vi "Rig - Editor.vi"(8 "Error IN":errorcluster) -> (0 "error out":errorcluster)   [LabVIEW 2018]
doc: "This VI allows the user to reprocess and reprint data sheets from previously run ESS test. User can search for vibe or thermal test for both actuators and controllers through this portal. Double click serial number from 'Available Data Files' listbox and press 'Print' to initiate report regeneration."
uses:
  controls/Rig Config Settings.ctl
  controls/Command IN_Recipe.ctl
  Globals/Global - Configuration Options.vi
panel:
  in  "Rename":bool
  in  "Exit":bool
  out "Rig Config File Name":string
  in  "Rig Settings":T1={"Rig Name"="", "Rig Room"="1.4", "Base Directory"="", "Computer IP Address"="", "Globals Name"="", "Treatmill Str"="", "cRIO Test Data Dir"=path "", "ai"="", "ao"="", "dio"="", "A_calib_str_row1"="", "A_calib_str_row2"="0", "A_calib_str_row3"="1.4", "Zero_V_str"="", "step_V"="", "Sample Freq"="", "ai_threshold"="", "run_speed_thresh"="", "speed_time_length"="", "wall ball gain"="", "max wall pos"="", "max cor width"="", "Trial Config Directory"=path "C:/Whisker Tester/Trials", "Randomize Trials?"=FALSE}
  in  "Save":bool
  in  "New":bool
  in  "Delete":bool
  in  "Rig File List":i32(listbox)
  in  "Refresh":bool
  out "Rig File Path":path
  in  "Functions":enum16{"Initialize", "Exit"}(ring)
  out "Rig Config Directory":path=path "C:/Data"
  # "Rig Configuration Screen"
  # "*click on rig file to view"
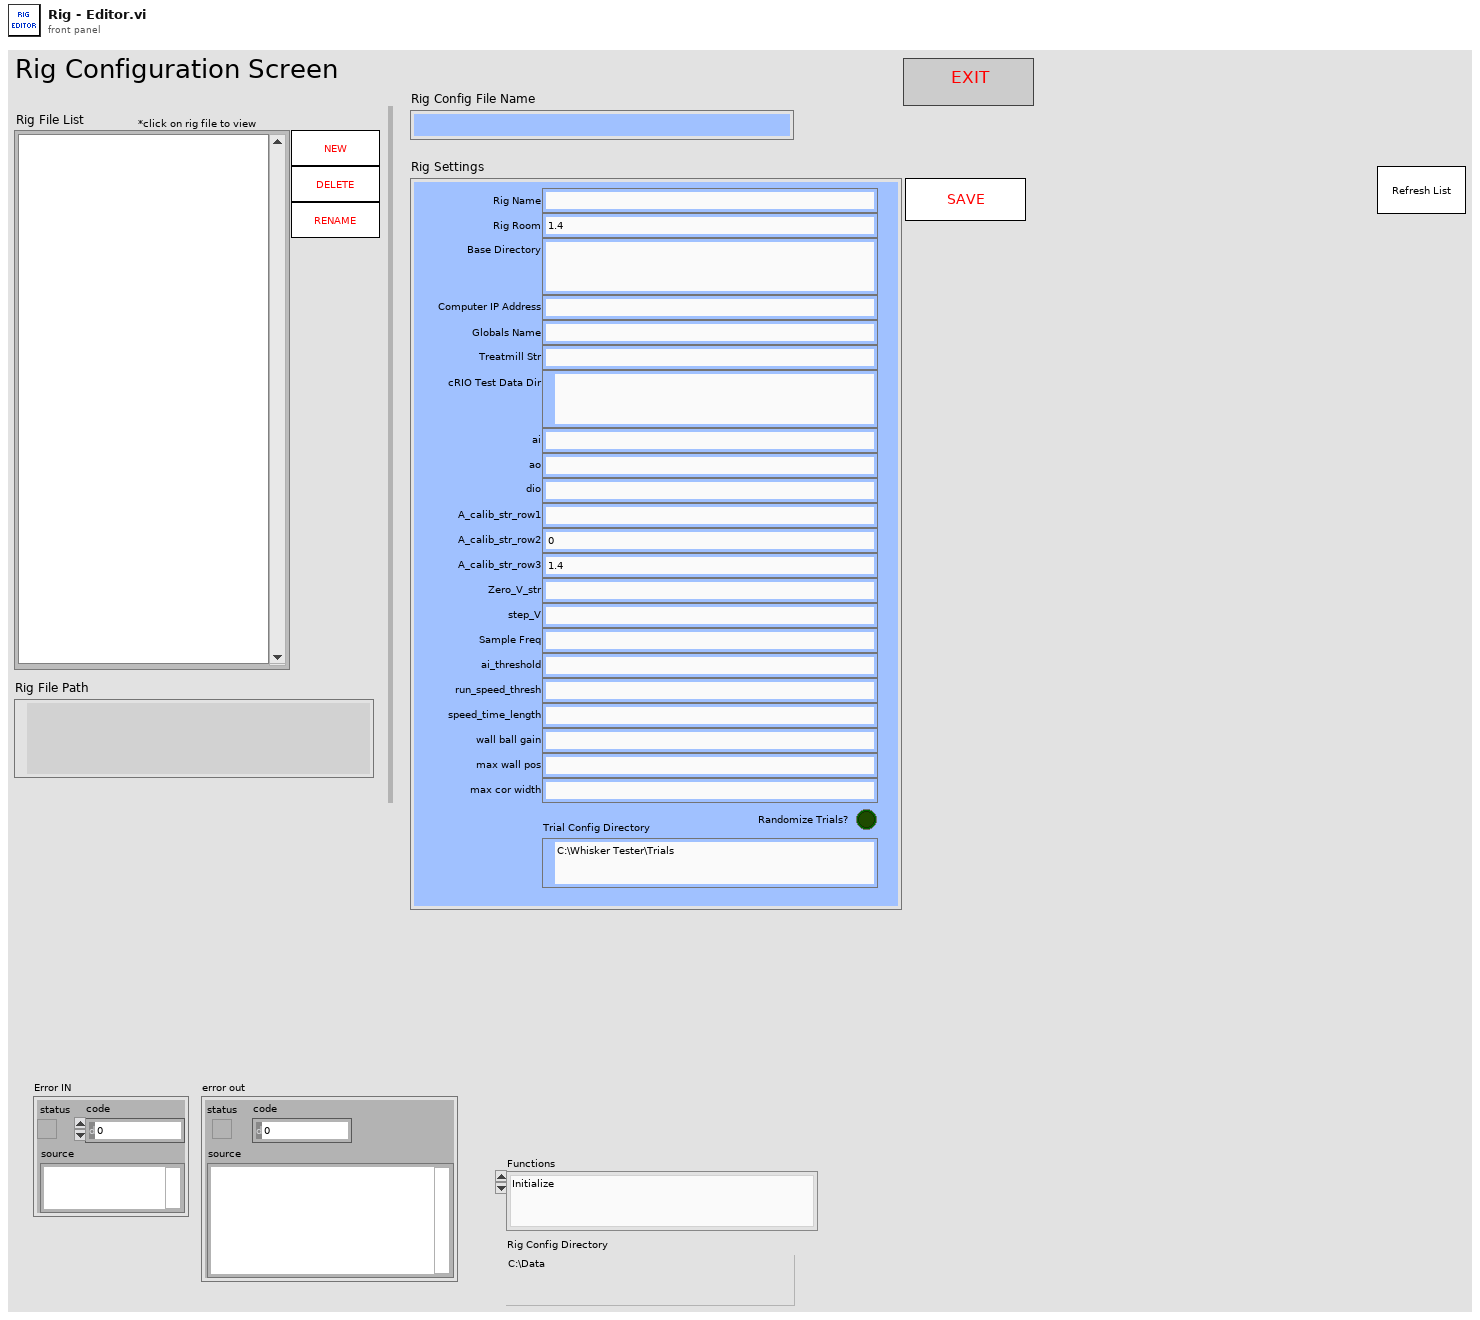
[diagram p1: front panel]
types:
  T1 = typedef "Rig Config Settings.ctl" = cluster{"Rig Name":string, "Rig Room":string, "Base Directory":string, "Computer IP Address":string, "Globals Name":string, "Treatmill Str":string, "cRIO Test Data Dir":path, "ai":string, "ao":string, "dio":string, "A_calib_str_row1":string, "A_calib_str_row2":string, "A_calib_str_row3":string, "Zero_V_str":string, "step_V":string, "Sample Freq":string, "ai_threshold":string, "run_speed_thresh":string, "speed_time_length":string, "wall ball gain":string, "max wall pos":string, "max cor width":string, "Trial Config Directory":path, "Randomize Trials?":bool}
  T2 = typedef "Command IN_Recipe.ctl" = enum16{"Save", "Load"}
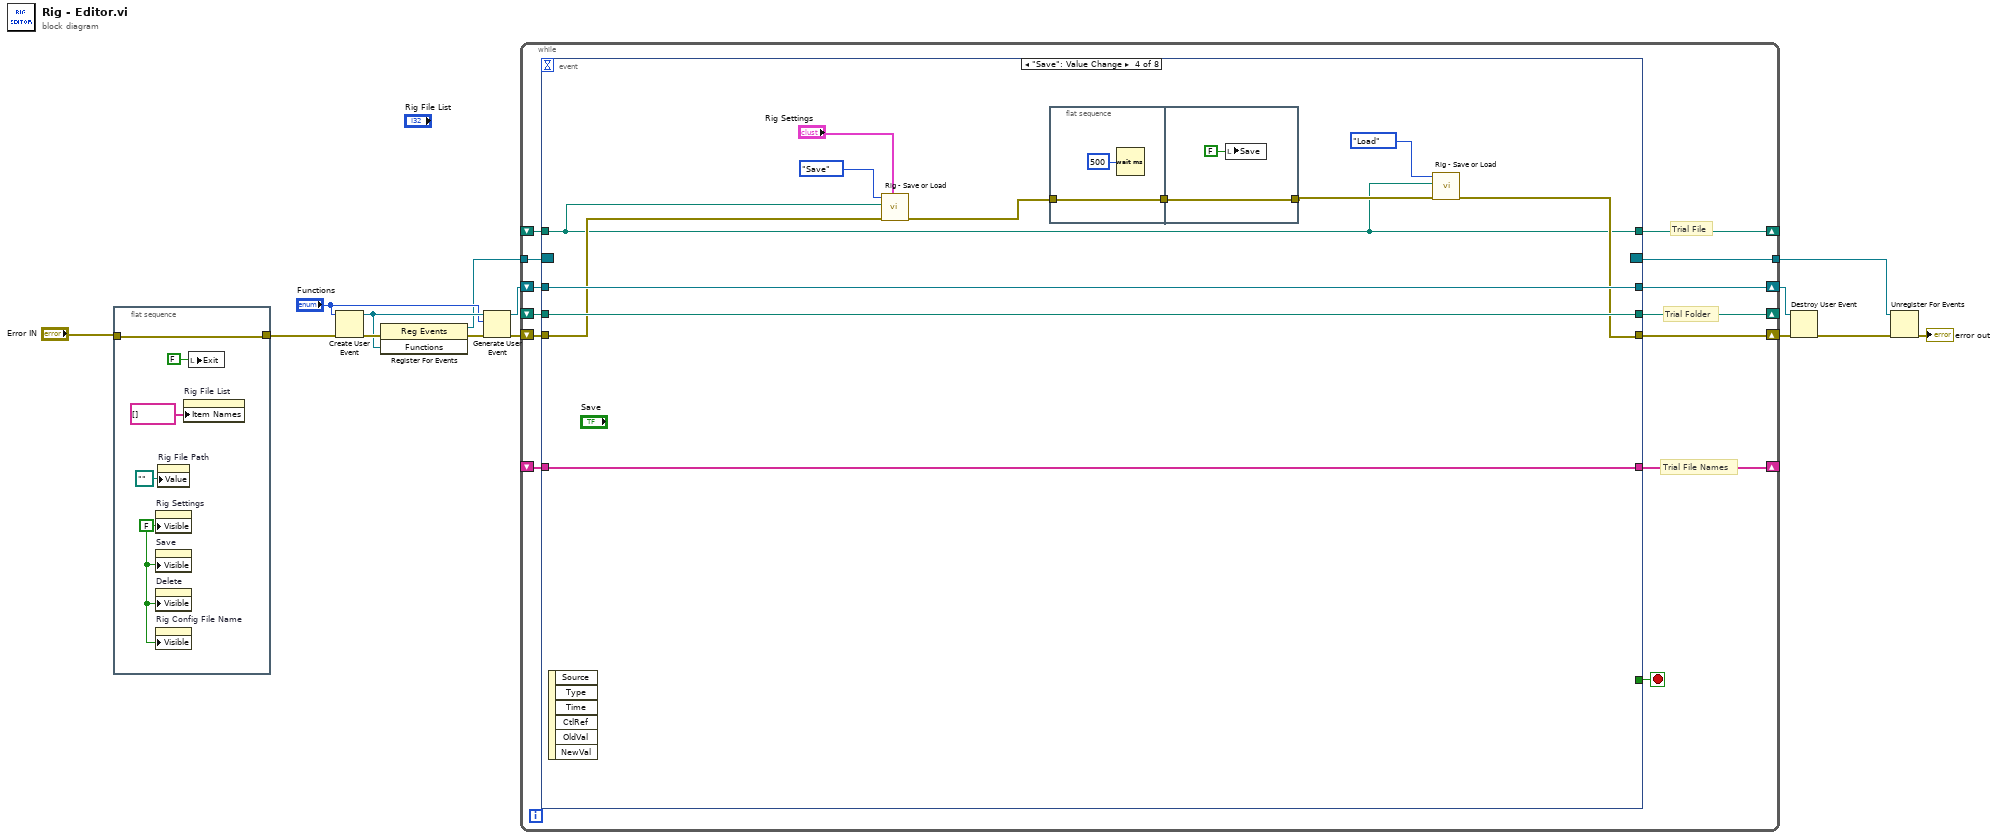
[diagram p0: block diagram]
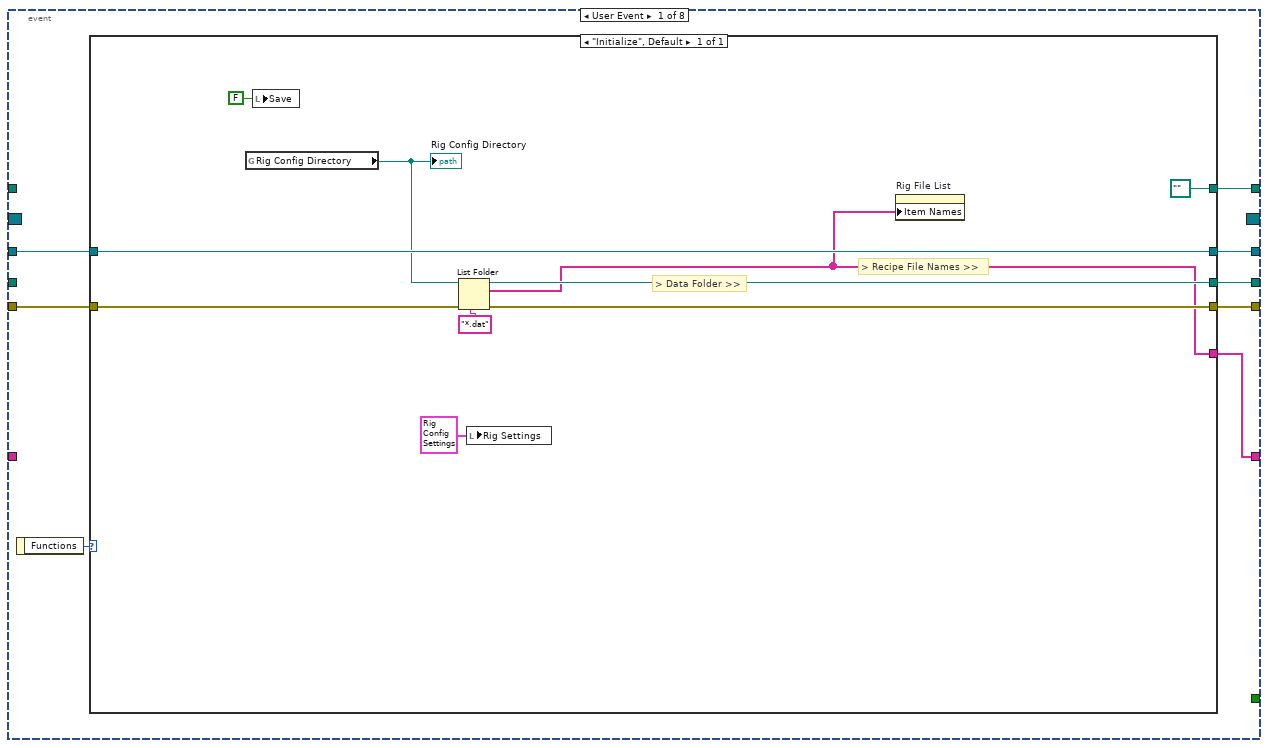
[diagram p2: hidden frame]
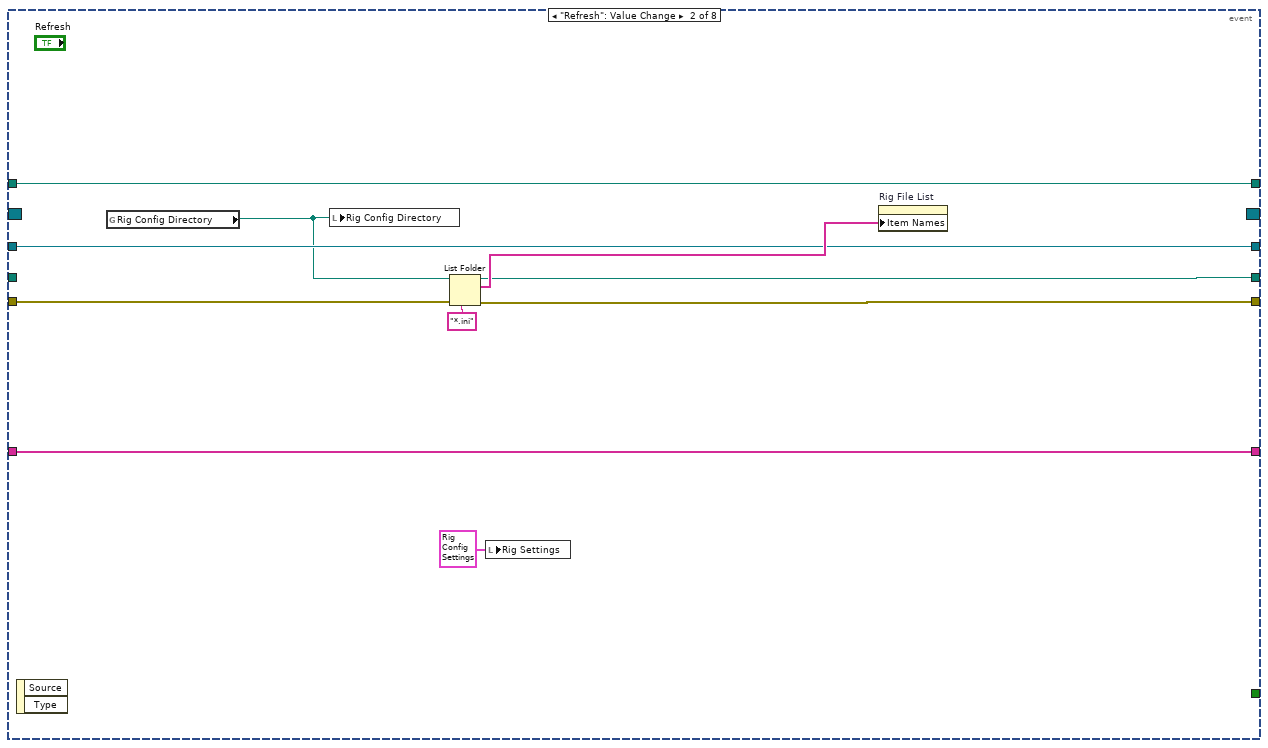
[diagram p3: hidden frame]
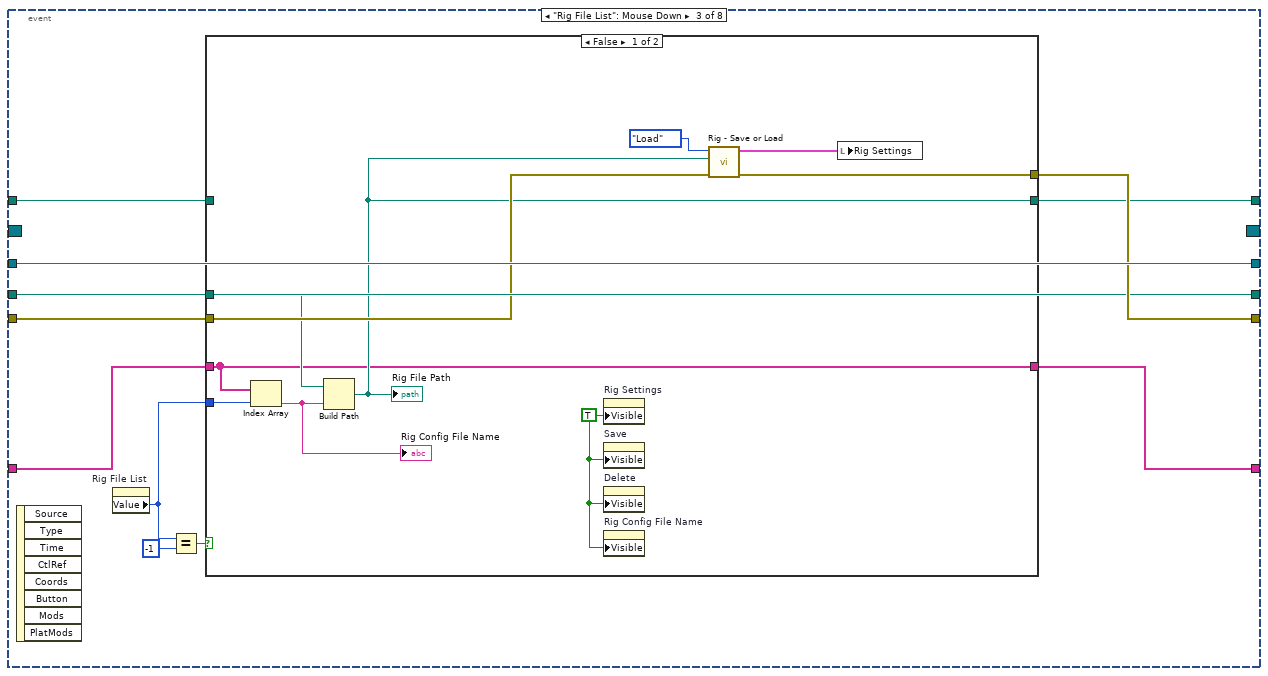
[diagram p4: hidden frame]
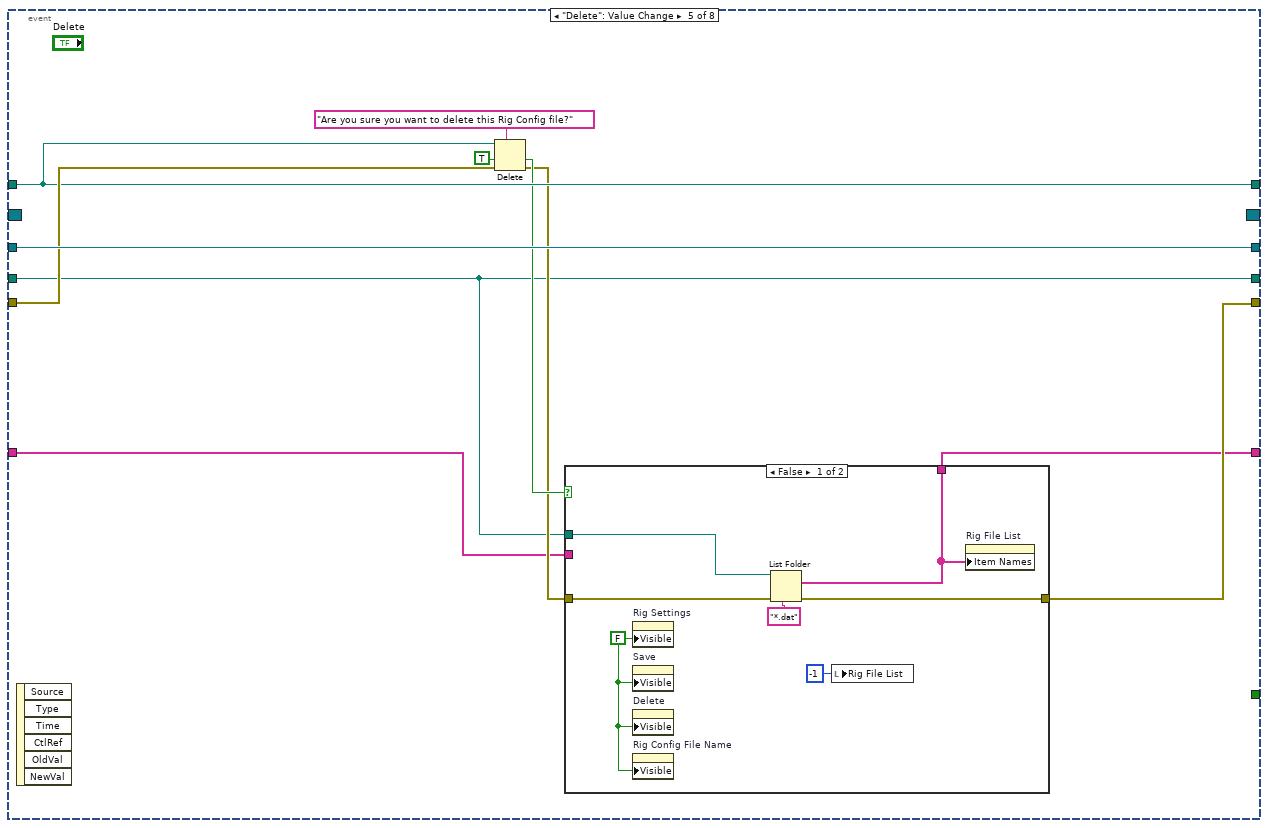
[diagram p6: hidden frame]
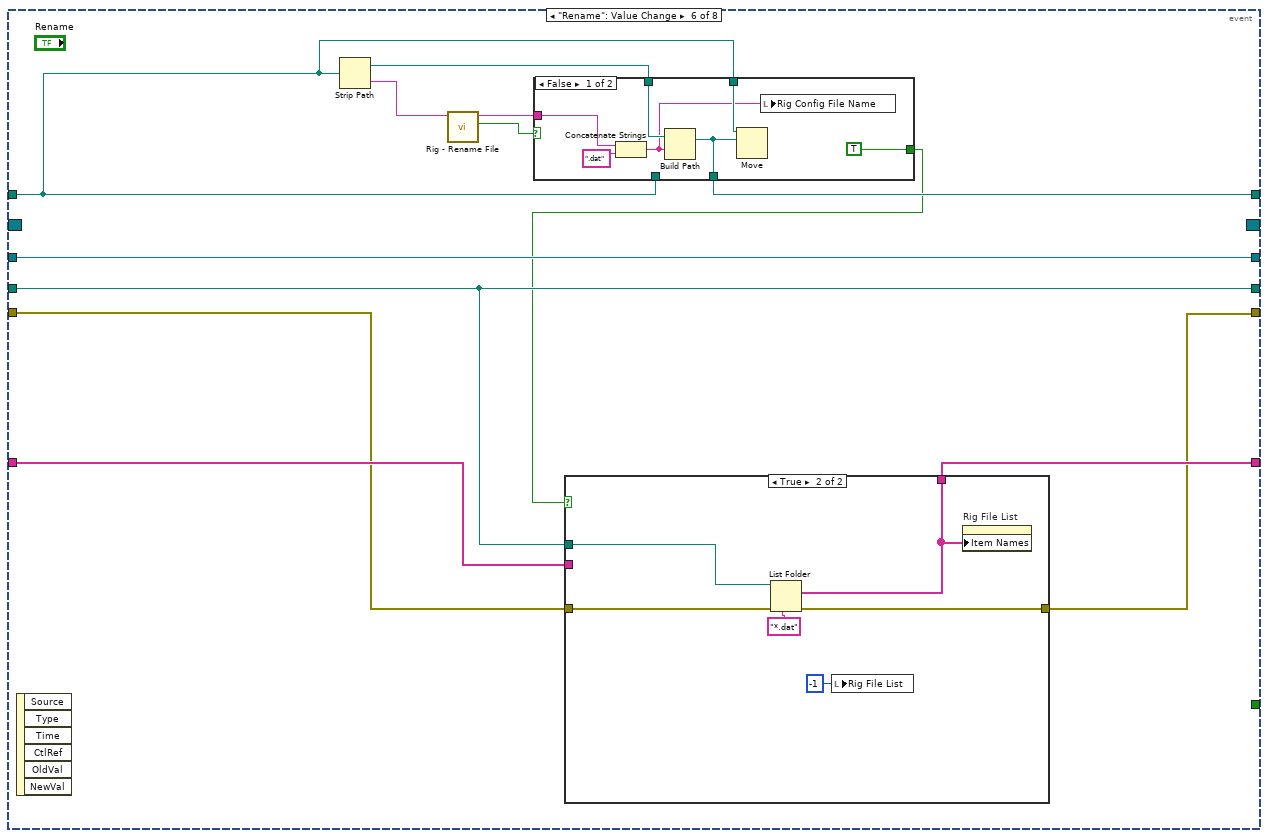
[diagram p8: hidden frame]
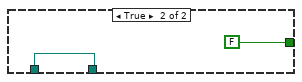
[diagram p9: hidden frame]
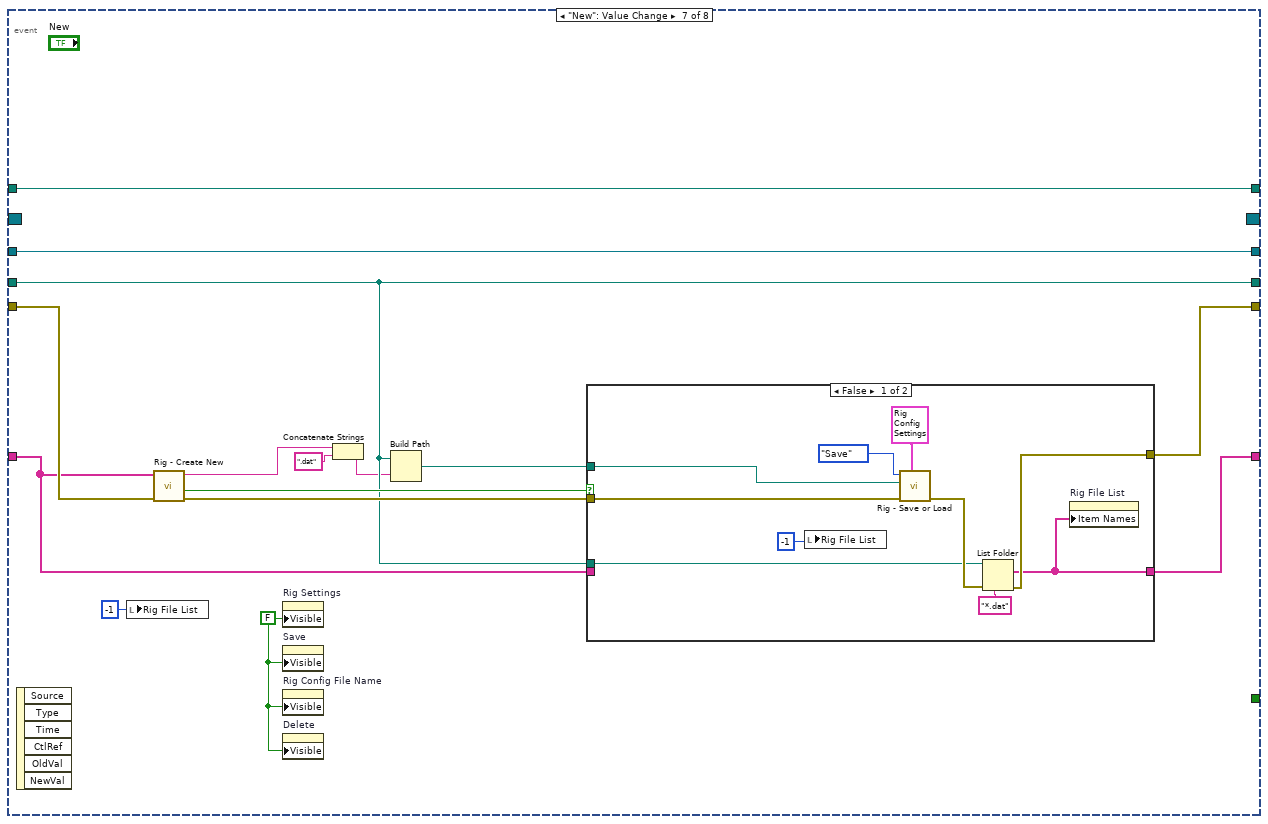
[diagram p11: hidden frame]
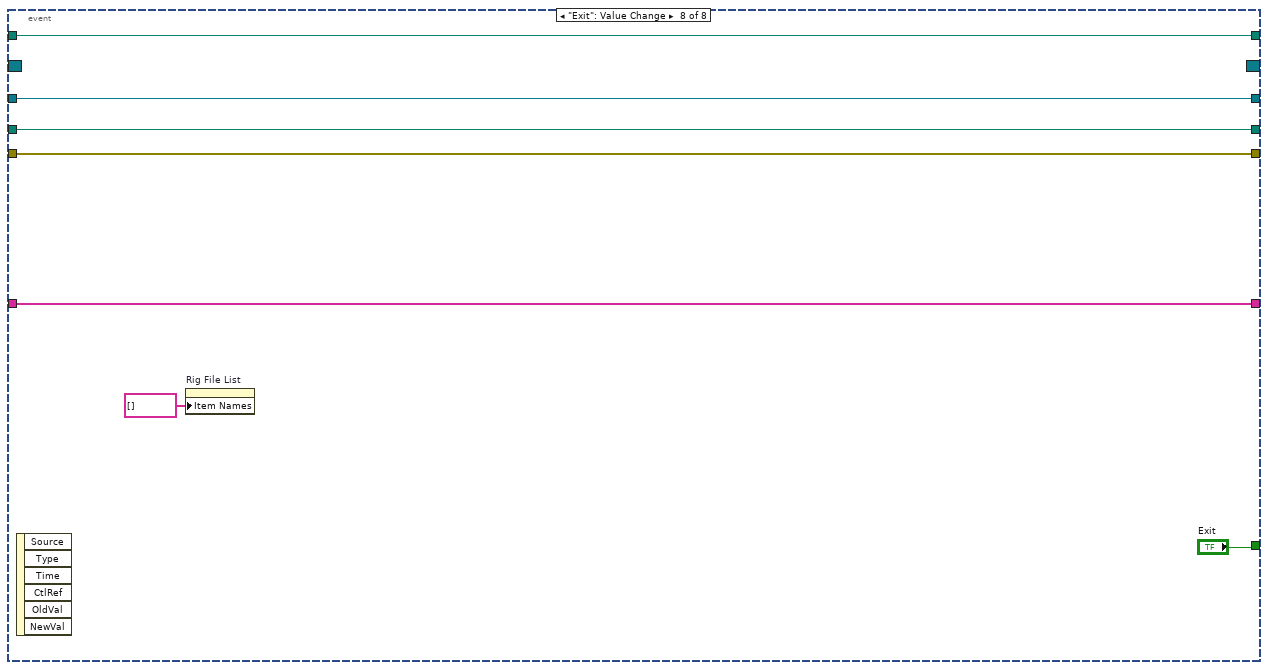
[diagram p13: hidden frame]
diagram:
  n1 = flat-sequence {
    tunnel: "Error IN" -> [w15]
    tunnel: [w15] -> w1
    frame #0 {
      w17 = FALSE ("Visible")
      n2 = property on="Rig Settings" class="Clust (strict)"("Visible"=w17) -> ()  [unwired: 2 in, 2 out]
      n3 = property on="Save" class="Bool (strict)"("Visible"=w17) -> ()  [unwired: 2 in, 2 out]
      n4 = property on="Delete" class="Bool"("Visible"=w17) -> ()  [unwired: 2 in, 2 out]
      n5 = property on="Rig Config File Name" class="Str"("Visible"=w17) -> ()  [unwired: 2 in, 2 out]
      n6 = property on="Rig File Path" class="Path"("Value"=path "" ("Data File Selected")) -> ()  [unwired: 2 in, 2 out]
      n7 = property on="Rig File List" class="LstBox (strict)"("Item Names"=string[] []) -> ()  [unwired: 2 in, 2 out]
      n8 = local write "Exit"(FALSE ("Exit")) -> ()
    }
  }
  n9 = Create User Event(user event datatype="Functions", error in=w1) -> (user event=w12:refnum<user-event>, error out=w14:errorcluster)
  n10 = register-events(error in=w14, w12) -> (reference out=w10:refnum<event-registration>, error out=w13:errorcluster)  [unwired: 1 in]
  n11 = Generate User Event(user event=w12, event data cluster="Functions", error in=w13) -> (user event out=w8:refnum<user-event>, error out=w9:errorcluster)  [unwired: 1 in]
  n12 = while {
    tunnel: w10 -> [w32]
    shift-right: [w30] -> w7
    shift-left: w9 -> [w31]
    shift-right: [w29] -> _
    shift-left: _ -> [w23]
    shift-right: [w28] -> w6
    shift-left: w8 -> [w27]
    tunnel: [w26] -> w4
    shift-right: [w25] -> _
    shift-left: _ -> [w24]
    shift-right: [w21] -> _
    shift-left: _ -> [w20]
    stop <- w22 stop-if-true
    # "Trial File"
    # "Trial Folder"
    # "Trial File Names"
    n13 = event shown="[3] \"Save\": Value Change" {
      selector: w32 -> [_ _ _ _ _ _ _ _]
      dyn-events: [_ _ _ _ _ _ _ _] -> w26
      timeout: _ -> [_ _ _ _ _ _ _ _]
      tunnel: w31 -> [w39 w57 w69 w93 w110 w122 w163 w182]
      tunnel: [w38 w56 w68 w88 w105 w121 w160 w182] -> w30
      tunnel: [w37 w55 w67 w94 w102 w130 w158 w181] -> w29
      tunnel: [w36 w54 w70 w95 w111 w133 w165 w183] -> w28
      tunnel: w27 -> [w35 w54 w70 w95 w111 w133 w165 w183]
      tunnel: [w34 w53 w61 w96 w104 w132 w154 w180] -> w25
      tunnel: w24 -> [_ w53 w71 w96 w103 w131 w151 w180]
      tunnel: w23 -> [_ _ w67 w94 w102 w130 w158 w181]
      tunnel: [_ _ _ _ _ _ _ "Exit"] -> w22
      tunnel: [w33 w60 w66 w85 w109 w124 w164 w184] -> w21
      tunnel: w20 -> [_ w60 w62 w85 w109 w125 w164 w184]
      event User Event {
        n14 = event-data() -> ("Functions"=w40:enum16{"Initialize", "Exit"})  [unwired: 1 in]
        n15 = case shown="\"Initialize\", Default" w40 {
          tunnel: w39 -> [w49]
          tunnel: [w48] -> w38
          tunnel: [w47] -> w37
          tunnel: [w46] -> w36
          tunnel: w35 -> [w46]
          tunnel: [w44] -> w34
          tunnel: [path "" ("appended path")] -> w33
          frame "Initialize", Default {
            # "> Recipe File Names >>"
            # "> Data Folder >>"
            n16 = global read "Global - Configuration Options.vi" "Rig Config Directory"() -> (w41:path)
            "Rig Config Directory" <- w41
            n17 = local write "Save"(FALSE ("Save")) -> ()
            n18 = List Folder(path=w41, pattern="*.dat", error in=w49) -> (path out=w47:path, filenames=w44:string[], error out=w48:errorcluster)  [unwired: 1 in, 1 out]
            n19 = local write "Rig Settings"(T1 {"Rig Name"="", "Rig Room"="1.4", "Base Directory"="", "Computer IP Address"="", "Globals Name"="", "Treatmill Str"="", "cRIO Test Data Dir"=path "", "ai"="", "ao"="", "dio"="", "A_calib_str_row1"="", "A_calib_str_row2"="0", "A_calib_str_row3"="1.4", "Zero_V_str"="", "step_V"="", "Sample Freq"="", "ai_threshold"="", "run_speed_thresh"="", "speed_time_length"="", "wall ball gain"="", "max wall pos"="", "max cor width"="", "Trial Config Directory"=path "C:/Whisker Tester/Trials", "Randomize Trials?"=FALSE} ("Rig Settings")) -> ()
            n20 = property on="Rig File List" class="LstBox (strict)"("Item Names"=w44) -> ()  [unwired: 2 in, 2 out]
          }
        }
      }
      event "Refresh": Value Change {
        n21 = event-data() -> ()  [unwired: 1 in, 2 out]
        n22 = global read "Global - Configuration Options.vi" "Rig Config Directory"() -> (w51:path)
        n23 = local write "Rig Config Directory"(w51) -> ()
        n24 = List Folder(path=w51, pattern="*.ini", error in=w57) -> (path out=w55:path, filenames=w58:string[], error out=w56:errorcluster)  [unwired: 1 in, 1 out]
        n25 = local write "Rig Settings"(T1 {"Rig Name"="", "Rig Room"="1.4", "Base Directory"="", "Computer IP Address"="", "Globals Name"="", "Treatmill Str"="", "cRIO Test Data Dir"=path "", "ai"="", "ao"="", "dio"="", "A_calib_str_row1"="", "A_calib_str_row2"="0", "A_calib_str_row3"="1.4", "Zero_V_str"="", "step_V"="", "Sample Freq"="", "ai_threshold"="", "run_speed_thresh"="", "speed_time_length"="", "wall ball gain"="", "max wall pos"="", "max cor width"="", "Trial Config Directory"=path "C:/Whisker Tester/Trials", "Randomize Trials?"=FALSE} ("Rig Settings")) -> ()
        n26 = property on="Rig File List" class="LstBox (strict)"("Item Names"=w58) -> ()  [unwired: 2 in, 2 out]
      }
      event "Rig File List": Mouse Down {
        n27 = event-data() -> ()  [unwired: 1 in, 8 out]
        n28 = property on="Rig File List" class="LstBox (strict)"() -> ("Value"=w64:i32)  [unwired: 2 in, 2 out]
        n29 = Equal?(x=w64, y=-1) -> (x = y?=w65:bool)
        n30 = case shown="False" w65 {
          tunnel: w71 -> [w74 w82]
          tunnel: w69 -> [w81 w84]
          tunnel: [w80 w84] -> w68
          tunnel: w67 -> [w79 _]
          tunnel: [w77 w83] -> w66
          tunnel: w64 -> [w75 _]
          tunnel: w62 -> [_ w83]
          tunnel: [w74 w82] -> w61
          frame False {
            w76 = TRUE ("Visible")
            n31 = Index Array(array=w74, index=w75) -> (element=w78:string)
            "Rig Config File Name" <- w78
            n32 = Build Path(base path=w79, name or relative path=w78) -> (appended path=w77:path)
            "Rig File Path" <- w77
            n33 = property on="Rig Settings" class="Clust (strict)"("Visible"=w76) -> ()  [unwired: 2 in, 2 out]
            n34 = property on="Save" class="Bool (strict)"("Visible"=w76) -> ()  [unwired: 2 in, 2 out]
            n35 = property on="Delete" class="Bool"("Visible"=w76) -> ()  [unwired: 2 in, 2 out]
            n36 = property on="Rig Config File Name" class="Str"("Visible"=w76) -> ()  [unwired: 2 in, 2 out]
            n37 = call "Rig - Save or Load.vi"("Error IN"=w81, "RigSave Path IN"=w77, "Command IN"=Command_IN_Recipe."Load") -> ("Error OUT"=w80:errorcluster, "Rig Settings OUT"=w72:T1)  [unwired: 7 in]
            n38 = local write "Rig Settings"(w72) -> ()
          }
          frame True {
          }
        }
      }
      event "Save": Value Change {
        n39 = event-data() -> ()  [unwired: 1 in, 6 out]
        n40 = call "Rig - Save or Load.vi"("Rig Settings IN"="Rig Settings", "Error IN"=w93, "RigSave Path IN"=w85, "Command IN"=Command_IN_Recipe."Save") -> ("Error OUT"=w92:errorcluster)  [unwired: 6 in, 1 out]
        n41 = flat-sequence {
          tunnel: w92 -> [w98]
          tunnel: [w98] -> w91
          tunnel: [w100] -> w87
          tunnel: w91 -> [w100]
          frame #0 {
            n42 = Wait (ms)(milliseconds to wait=u32 500) -> ()  [unwired: 1 out]
          }
          frame #1 {
            n43 = local write "Save"(FALSE ("Save")) -> ()
          }
        }
        n44 = call "Rig - Save or Load.vi"("Error IN"=w87, "RigSave Path IN"=w85, "Command IN"=Command_IN_Recipe."Load") -> ("Error OUT"=w88:errorcluster)  [unwired: 7 in, 1 out]
      }
      event "Delete": Value Change {
        n45 = event-data() -> ()  [unwired: 1 in, 6 out]
        n46 = Delete(prompt (Delete)="Are you sure you want to delete this Rig Config file?", path (use dialog)=w109, confirm (F)=TRUE, error in=w110) -> (cancelled=w107:bool, error out=w106:errorcluster)  [unwired: 1 in, 1 out]
        n47 = case shown="False" w107 {
          tunnel: w106 -> [w117 w120]
          tunnel: [w116 w120] -> w105
          tunnel: [w115 w119] -> w104
          tunnel: w103 -> [_ w119]
          tunnel: w102 -> [w114 _]
          frame False {
            w112 = FALSE ("Visible")
            n48 = property on="Rig Settings" class="Clust (strict)"("Visible"=w112) -> ()  [unwired: 2 in, 2 out]
            n49 = property on="Save" class="Bool (strict)"("Visible"=w112) -> ()  [unwired: 2 in, 2 out]
            n50 = property on="Delete" class="Bool"("Visible"=w112) -> ()  [unwired: 2 in, 2 out]
            n51 = property on="Rig Config File Name" class="Str"("Visible"=w112) -> ()  [unwired: 2 in, 2 out]
            n52 = List Folder(path=w114, pattern="*.dat", error in=w117) -> (filenames=w115:string[], error out=w116:errorcluster)  [unwired: 1 in, 2 out]
            n53 = local write "Rig File List"(-1 ("Recipe List")) -> ()
            n54 = property on="Rig File List" class="LstBox (strict)"("Item Names"=w115) -> ()  [unwired: 2 in, 2 out]
          }
          frame True {
          }
        }
      }
      event "Rename": Value Change {
        n55 = event-data() -> ()  [unwired: 1 in, 6 out]
        n56 = Strip Path(path=w125) -> (stripped path=w129:path, name=w128:string)
        n57 = call "Rig - Rename File.vi"("Current File Name"=w128) -> ("Cancel OUT"=w126:bool, "Enter New File Name OUT"=w127:string)  [unwired: 9 in]
        n58 = case shown="False" w126 {
          tunnel: w129 -> [w139 _]
          tunnel: w125 -> [w138 _]
          tunnel: w127 -> [w137 _]
          tunnel: w125 -> [_ w142]
          tunnel: [w136 w142] -> w124
          tunnel: [TRUE FALSE] -> w123
          frame False {
            n59 = Concatenate Strings(w137, ".dat") -> (w134:string)
            n60 = Build Path(base path=w139, name or relative path=w134) -> (appended path=w136:path)
            n61 = Move(source path=w138, 10:w136) -> ()  [unwired: 3 in, 3 out]
            n62 = local write "Rig Config File Name"(w134) -> ()
          }
          frame True {
          }
        }
        n63 = case shown="True" w123 {
          tunnel: w122 -> [w144 w149]
          tunnel: [w144 w148] -> w121
          tunnel: [w143 w147] -> w132
          tunnel: w131 -> [w143 _]
          tunnel: w130 -> [_ w146]
          frame False {
          }
          frame True {
            n64 = List Folder(path=w146, pattern="*.dat", error in=w149) -> (filenames=w147:string[], error out=w148:errorcluster)  [unwired: 1 in, 2 out]
            n65 = local write "Rig File List"(-1 ("Recipe List")) -> ()
            n66 = property on="Rig File List" class="LstBox (strict)"("Item Names"=w147) -> ()  [unwired: 2 in, 2 out]
          }
        }
      }
      event "New": Value Change {
        w153 = FALSE ("Visible")
        n67 = event-data() -> ()  [unwired: 1 in, 6 out]
        n68 = local write "Rig File List"(-1 ("Recipe List")) -> ()
        n69 = call "Rig - Create New.vi"("Error IN"=w163, "Existing Rig Config Names"=w151) -> ("Error OUT"=w161:errorcluster, "Cancel OUT"=w162:bool, "Enter New Rig Config File Name OUT"=w156:string)  [unwired: 7 in]
        n70 = property on="Rig Settings" class="Clust (strict)"("Visible"=w153) -> ()  [unwired: 2 in, 2 out]
        n71 = property on="Save" class="Bool (strict)"("Visible"=w153) -> ()  [unwired: 2 in, 2 out]
        n72 = property on="Rig Config File Name" class="Str"("Visible"=w153) -> ()  [unwired: 2 in, 2 out]
        n73 = property on="Delete" class="Bool"("Visible"=w153) -> ()  [unwired: 2 in, 2 out]
        n74 = Concatenate Strings(w156, ".dat" ("string")) -> (w155:string)
        n75 = Build Path(base path=w158, name or relative path=w155) -> (appended path=w159:path)
        n76 = case shown="False" w162 {
          tunnel: w161 -> [w175 w177]
          tunnel: [w170 w177] -> w160
          tunnel: w159 -> [w173 _]
          tunnel: w158 -> [w169 _]
          tunnel: [w168 w176] -> w154
          tunnel: w151 -> [_ w176]
          frame False {
            n77 = local write "Rig File List"(-1 ("Recipe List")) -> ()
            n78 = call "Rig - Save or Load.vi"("Rig Settings IN"=T1 {"Rig Name"="", "Rig Room"="1.4", "Base Directory"="", "Computer IP Address"="", "Globals Name"="", "Treatmill Str"="", "cRIO Test Data Dir"=path "", "ai"="", "ao"="", "dio"="", "A_calib_str_row1"="", "A_calib_str_row2"="0", "A_calib_str_row3"="1.4", "Zero_V_str"="", "step_V"="", "Sample Freq"="", "ai_threshold"="", "run_speed_thresh"="", "speed_time_length"="", "wall ball gain"="", "max wall pos"="", "max cor width"="", "Trial Config Directory"=path "C:/Whisker Tester/Trials", "Randomize Trials?"=FALSE}, "Error IN"=w175, "RigSave Path IN"=w173, "Command IN"=Command_IN_Recipe."Save") -> ("Error OUT"=w171:errorcluster)  [unwired: 6 in, 1 out]
            n79 = List Folder(path=w169, pattern="*.dat", error in=w171) -> (filenames=w168:string[], error out=w170:errorcluster)  [unwired: 1 in, 2 out]
            n80 = property on="Rig File List" class="LstBox (strict)"("Item Names"=w168) -> ()  [unwired: 2 in, 2 out]
          }
          frame True {
          }
        }
      }
      event "Exit": Value Change {
        n81 = event-data() -> ()  [unwired: 1 in, 6 out]
        n82 = property on="Rig File List" class="LstBox (strict)"("Item Names"=string[] []) -> ()  [unwired: 2 in, 2 out]
      }
    }
  }
  n83 = Destroy User Event(user event=w6, error in=w7) -> (error out=w5:errorcluster)
  n84 = Unregister For Events(event registration refnum=w4, error in=w5) -> (error out=→"error out":errorcluster)
